vi "Read Destination.vi"(8 "error in (no error)":errorcluster, 11 "Job.SingleFileCopy in":refnum<class "Job.SingleFileCopy.lvclass">) -> (0 "error out":errorcluster, 2 "Destination":path, 3 "Job.SingleFileCopy out":refnum<class "Job.SingleFileCopy.lvclass">)   [LabVIEW 2013, in "Job.SingleFileCopy.lvclass"]
uses:
  Job.SingleFileCopy.lvclass
  Job.SingleFileCopy.lvclass/Job.SingleFileCopy.ctl
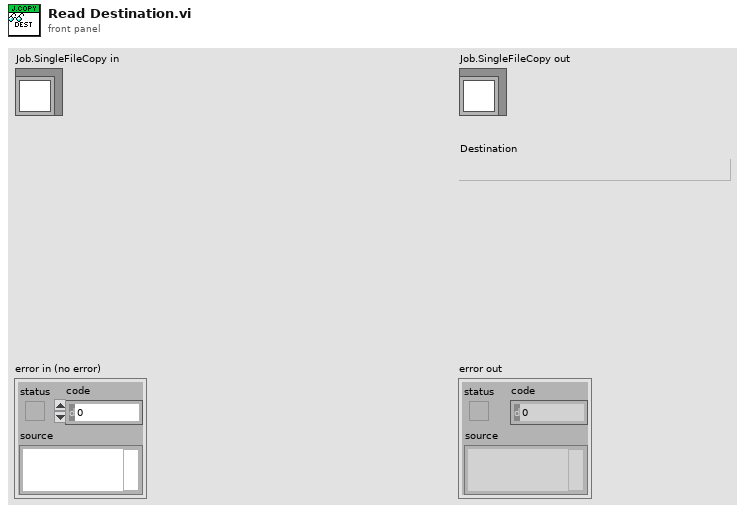
[diagram p1: front panel]
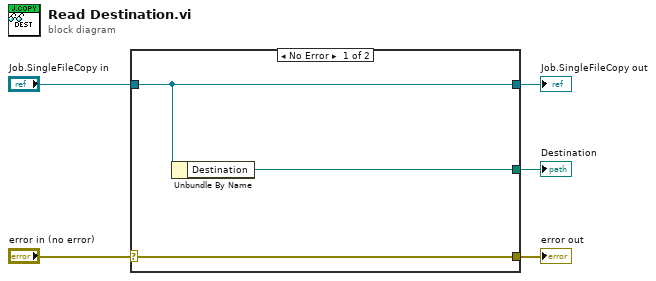
[diagram p0: block diagram]
diagram:
  n1 = case shown="No Error" "error in (no error)" {
    selector: "error in (no error)" -> [w8 w9]
    tunnel: [w8 w9] -> w4
    tunnel: [w7 w10] -> w2
    tunnel: "Job.SingleFileCopy in" -> [w7 w10]
    tunnel: [w6 _] -> w1
    frame No Error {
      n2 = Unbundle By Name(w7) -> ("Destination"=w6:path)
    }
    frame Error {
    }
  }
  "error out" <- w4
  "Job.SingleFileCopy out" <- w2
  "Destination" <- w1
